vi "Clean Up References.vi"(8 "error in (no error)":errorcluster, 11 "Panel Form Controller in":refnum<class "Panel Form Controller.lvclass">) -> (0 "error out":errorcluster, 3 "Panel Form Controller out":refnum<class "Panel Form Controller.lvclass">)   [LabVIEW 2020, in "Panel Form Controller.lvlib" / "Panel Form Controller.lvclass"]
uses:
  Panel Form Controller.lvclass
  Panel Form Controller.lvclass/Panel Form Controller.ctl
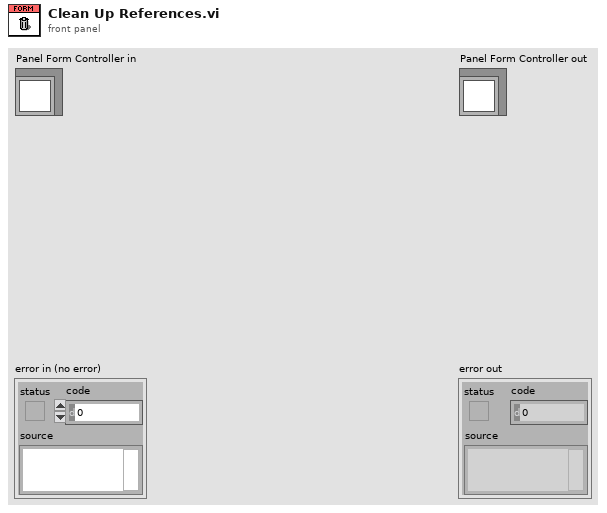
[diagram p1: front panel]
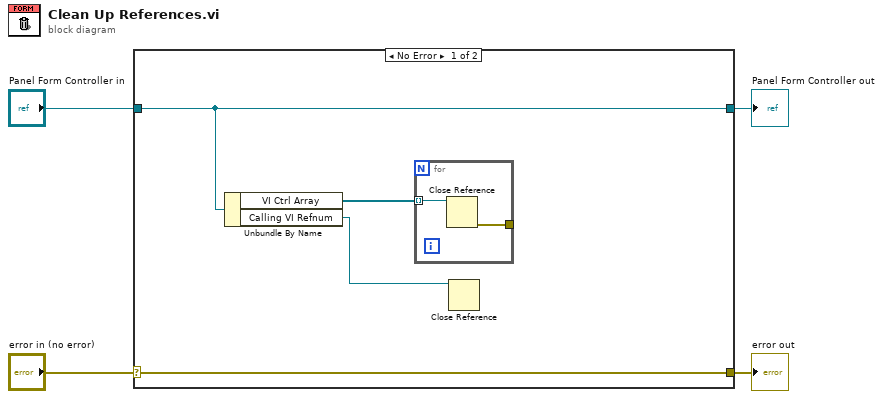
[diagram p0: block diagram]
diagram:
  n1 = case shown="No Error" "error in (no error)" {
    selector: "error in (no error)" -> [w8 w12]
    tunnel: [w8 w12] -> w3
    tunnel: [w7 w11] -> w1
    tunnel: "Panel Form Controller in" -> [w7 w11]
    frame No Error {
      n2 = Unbundle By Name(w7) -> ("VI Ctrl Array"=w6:refnum<vi>[], "Calling VI Refnum"=w5:refnum<vi>)
      n3 = for {
        tunnel: w6 -> [w10] mode=indexing
        tunnel: [w9] -> _
        n4 = Close Reference(reference=w10) -> (error out=w9:errorcluster)  [unwired: 1 in]
      }
      n5 = Close Reference(reference=w5) -> ()  [unwired: 1 in, 1 out]
    }
    frame Error {
    }
  }
  "error out" <- w3
  "Panel Form Controller out" <- w1
